vi "WriteSetpoint.vi"(9 "SetPoint":sgl, 10 "Device Data":T1 {"IDS" format="%.0x"; "IDL" format="%.0x"; "IDM" format="%.0x"; "IDH" format="%.0x"}) -> (1 "Message":string, 2 "Function Output Comment":string, 3 "Device Data OUT":T1 {"IDS" format="%.0x"; "IDL" format="%.0x"; "IDM" format="%.0x"; "IDH" format="%.0x"})   [LabVIEW 2019]
uses:
  Device Data.ctl
  164J027_AD/Brooks DLL 1.0.1.0 32bit/Brooks DLL 1.0.1.0 Release 10032016/S Protocol/BrooksDLL.dll
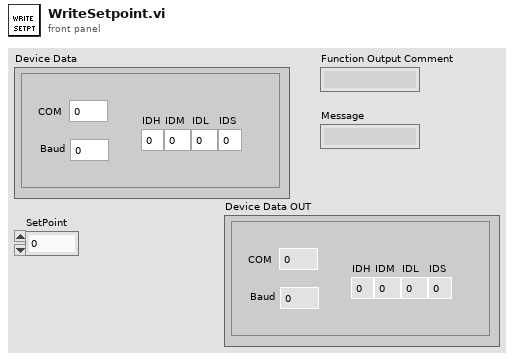
[diagram p1: front panel]
types:
  T1 = typedef "Device Data.ctl" = cluster{"COM":i32, "Baud":i32, "IDH":u8, "IDM":u8, "IDL":u8, "IDS":u8}
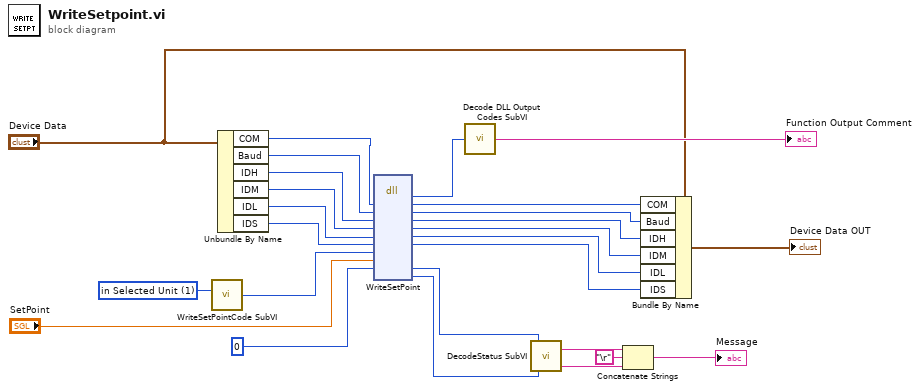
[diagram p0: block diagram]
diagram:
  w9 = u16 1 items=["in %", "in Selected Unit"] ("SetPointCode")
  n1 = call "WriteSetPointCode SubVI.vi"("SetPointCode 2"=w9) -> ("SetPointCode"=w10:u8)
  n2 = Unbundle By Name("Device Data") -> ("COM"=w21:i32, "Baud"=w22:i32, "IDH"=w26:u8, "IDM"=w25:u8, "IDL"=w24:u8, "IDS"=w23:u8)
  n3 = dll-call lib="G:/Developpement_de_Programmes/Programmes/Controle de pression/164J027_AD/Brooks DLL 1.0.1.0 32bit/Brooks DLL 1.0.1.0 Release 10032016/S Protocol/BrooksDLL.dll" fn="WriteSetPoint"("COM"=w21, "Baud"=w22, "IDH"=w26, "IDM"=w25, "IDL"=w24, "IDS"=w23, "SetPointCode"=w10, "SetPoint"="SetPoint", "S1"=u8 0) -> ("return type"=w13:i32, "COM"=w7:i32, "Baud"=w6:i32, "IDH"=w5:u8, "IDM"=w4:u8, "IDL"=w3:u8, "IDS"=w2:u8, "S1"=w11:u8, "S2"=w12:u8)  [unwired: 6 in, 2 out]
  n4 = call "Decode DLL Output Codes SubVI.vi"("Numeric"=w13) -> ("Function Output Comment"=→"Function Output Comment":string)
  n5 = call "DecodeStatus SubVI.vi"("S2"=w12, "S1"=w11) -> ("S2 String"=w19:string, "S1 String"=w20:string)
  n6 = Concatenate Strings(w20, "\r" ("string"), w19) -> (→"Message":string)
  n7 = Bundle By Name(cluster="Device Data", "COM"=w7, "Baud"=w6, "IDH"=w5, "IDM"=w4, "IDL"=w3, "IDS"=w2) -> (→"Device Data OUT":T1)
